vi "Cross_Correlation_slip.vi"() -> (5 "Plug in titles":string[](array[string]), 7 "Plug in values":string[](array[string]))   [LabVIEW 2010]
uses:
  Globals/Meas_global.vi
  Globals/Plug_in_data_global.vi
panel:
  out "Slip (ms)":dbl format="%.2f"
  in  "Slide":i32(slide) scale=-10.0..10.0
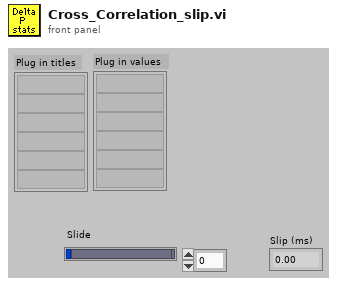
[diagram p1: front panel]
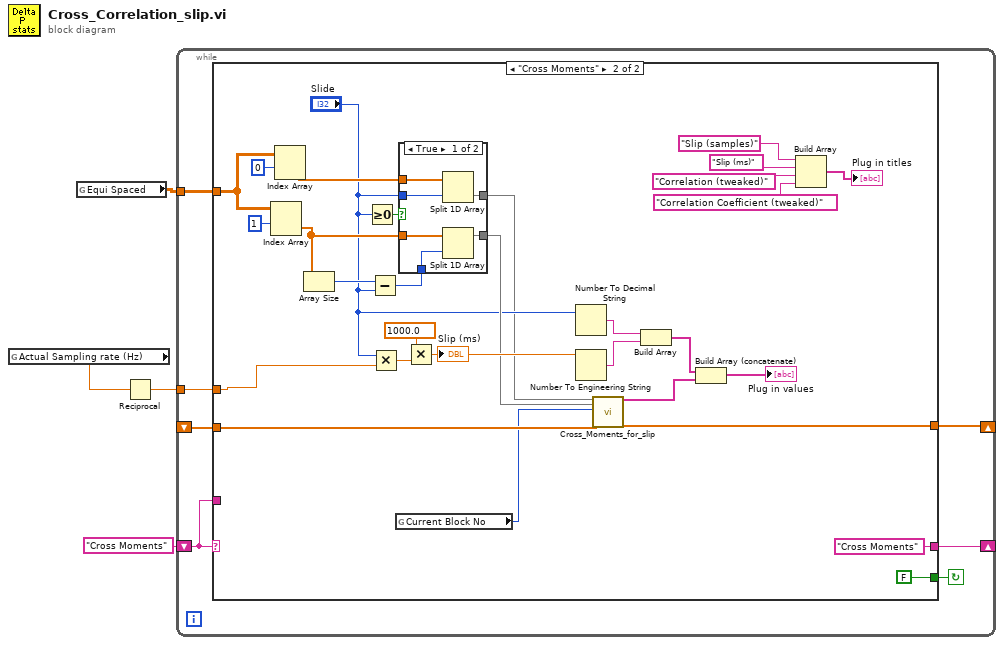
[diagram p0: block diagram]
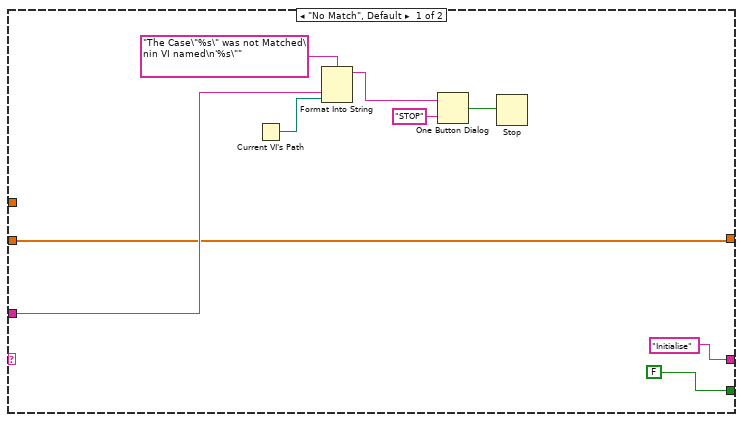
[diagram p2: hidden frame]
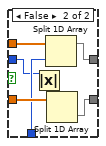
[diagram p3: hidden frame]
diagram:
  n1 = global read "Meas_global.vi" "Actual Sampling rate (Hz)"() -> (w2:dbl)
  n2 = global read "Plug_in_data_global.vi" "Equi Spaced"() -> (w1:dbl[][])
  n3 = Reciprocal(x=w2) -> (1/x=w3:dbl)
  n4 = while {
    shift-left: "Cross Moments" -> [w9]
    shift-right: [w10] -> _
    tunnel: w3 -> [w8]
    shift-right: [w7] -> _
    shift-left: _ -> [w6]
    tunnel: w1 -> [w5]
    stop <- w11 continue-if-true
    n5 = case shown="\"Cross Moments\"" w9 {
      tunnel: [FALSE FALSE] -> w11
      tunnel: ["Initialise" "Cross Moments"] -> w10
      tunnel: w9 -> [w15 _]
      tunnel: w8 -> [_ w30]
      tunnel: [w12 w45] -> w7
      tunnel: w6 -> [w12 w44]
      tunnel: w5 -> [_ w25]
      frame "No Match", Default {
        n6 = Current VI's Path() -> (path=w14:path)
        n7 = Format Into String(format string="The Case\"%s\" was not Matched\nin VI named\n'%s\"" ("Format String"), w15, w14) -> (resulting string=w18:string)  [unwired: 2 in, 1 out]
        n8 = One Button Dialog(message=w18, button name ("OK")="STOP") -> (true=w16:bool)
        n9 = Stop(stop? (T)=w16) -> ()
      }
      frame "Cross Moments" {
        n10 = Index Array(array=w25, index (row)=1) -> (element=w39:dbl[])  [unwired: 1 in]
        n11 = Index Array(array=w25, index (row)=0) -> (element=w40:dbl[])  [unwired: 1 in]
        n12 = Array Size(array=w39) -> (size(s)=w38:i32)
        n13 = Greater Or Equal To 0?(x="Slide") -> (x >= 0?=w23:bool)
        n14 = Subtract(x=w38, y="Slide") -> (x-y=w37:i32)
        n15 = Multiply(x="Slide", y=w30) -> (x*y=w29:dbl)
        n16 = global read "Meas_global.vi" "Current Block No"() -> (w41:i32)
        n17 = case shown="True" w23 {
          tunnel: w40 -> [w56 w63]
          tunnel: w39 -> [w55 w62]
          tunnel: w37 -> [w54 w61]
          tunnel: "Slide" -> [w53 w60]
          tunnel: [w52 w59] -> w21
          tunnel: [w51 w58] -> w24
          frame True {
            n18 = Split 1D Array(array=w56, index=w53) -> (second subarray=w52:dbl[])  [unwired: 1 out]
            n19 = Split 1D Array(array=w55, index=w54) -> (first subarray=w51:dbl[])  [unwired: 1 out]
          }
          frame False {
            n20 = Absolute Value(x=w60) -> (abs(x)=w57:i32)
            n21 = Split 1D Array(array=w63, index=w61) -> (first subarray=w59:dbl[])  [unwired: 1 out]
            n22 = Split 1D Array(array=w62, index=w57) -> (second subarray=w58:dbl[])  [unwired: 1 out]
          }
        }
        n23 = Multiply(x=1000.0, y=w29) -> (x*y=w27:dbl)
        "Slip (ms)" <- w27
        n24 = Number To Decimal String(number="Slide") -> (decimal integer string=w32:string)  [unwired: 1 out]
        n25 = Number To Engineering String(4:w27) -> (0:w26:string)  [unwired: 3 out]
        n26 = call "Cross_Moments_for_slip.vi"("U"=w21, "W"=w24, "Block No"=w41, "Shift in"=w44) -> ("Correlations Only"=w33:string[], "Shift out"=w45:dbl[])  [unwired: 14 out]
        n27 = Build Array(w32, w26) -> (w31:string[])
        n28 = Build Array (concatenate)(w31, w33) -> (→"Plug in values":string[])
        n29 = Build Array("Slip (samples)" ("element"), "Slip (ms)" ("element"), "Correlation (tweaked)", "Correlation Coefficient (tweaked)") -> (→"Plug in titles":string[])
      }
    }
  }
